vi "Get DDGIOC Pulses.vi"(8 "error in (no error)":errorcluster, 11 "pulses":i32) -> (0 "error out":errorcluster, 2 "function return":u32, 3 "pulses out":i32)   [LabVIEW 2014, in "atmcd32d.lvlib"]
doc: "unsigned int WINAPI GetDDGIOCPulses(int * pulses);"
uses:
  atmcd32d.lvlib
  atmcd32d.dll
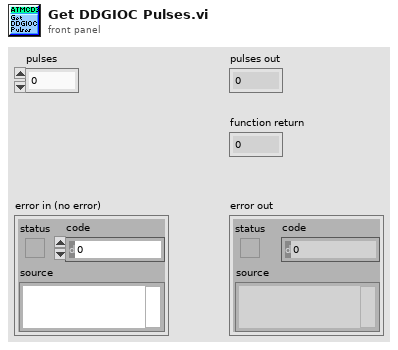
[diagram p1: front panel]
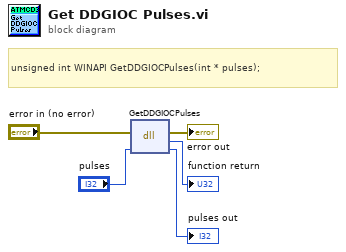
[diagram p0: block diagram]
diagram:
  # "unsigned int WINAPI GetDDGIOCPulses(int * pulses);"
  n1 = dll-call lib="C:/Users/Bakir/Documents/Lambda2-Testing/lib/Andorlib/atmcd32d.*" fn="GetDDGIOCPulses"(error in="error in (no error)", "pulses"="pulses") -> (error out=→"error out":errorcluster, →"function return":u32, "pulses"=→"pulses out":i32)  [unwired: 2 in, 1 out]
